vi "Rect Edit.vi"() -> ()   [LabVIEW 2019]
uses:
  Classes/Settings/Rectangle Settings/Rectangle Settings.lvclass/Rectangle Settings.ctl
  typedefs/Schedule Types/Schedule--Constant.ctl
  Classes/Settings/ObjectSettings/ObjectSettings.lvclass/ObjectSettings.ctl
  Classes/Settings/Setting Database/Setting Database.lvclass
  Classes/Settings/Rectangle Settings/Rectangle Settings.lvclass
  C:/Users/Albro/Documents/GitHub/AFM-Lithography/lvsrc/Classes/Settings/ObjectSettings/ObjectSettings.lvclass
  Classes/Settings/Setting Database/Typedefs/PrivateEvents--Setting Database.SetDefaultRectangle.ctl
  Classes/Settings/Setting Database/Typedefs/PrivateEvents--Setting Database.CopyActiveRectangleToAll.ctl
  <vilib>/JKI/JKI SMO/SMO/SMO.lvclass
  Classes/Settings/Rectangle Settings/Accessors/Write Fill Spacing.vi
  Classes/Settings/ObjectSettings/Accessors/Read Voltage Settings.vi
  Classes/Settings/ObjectSettings/Accessors/Read Speed Settings.vi
  Classes/Settings/ObjectSettings/Accessors/Write Resistance.vi
  Classes/Settings/ObjectSettings/Accessors/Write Speed Schedule.vi
  Classes/Settings/ObjectSettings/Accessors/Write Voltage Schedule.vi
  Classes/Settings/ObjectSettings/Accessors/Write Direction.vi
  Classes/Settings/ObjectSettings/Accessors/Write Enabled.vi
  Classes/Settings/Rectangle Settings/Accessors/Write Fill Orientation.vi
  Classes/Settings/ObjectSettings/Accessors/Read Enabled.vi
  Classes/Settings/ObjectSettings/Accessors/Read Direction.vi
  Classes/Settings/Rectangle Settings/Accessors/Read Fill Orientation.vi
  Classes/Settings/Rectangle Settings/Accessors/Read Fill Spacing.vi
  Classes/Settings/ObjectSettings/Accessors/Read Speed Schedule.vi
  Classes/Settings/ObjectSettings/Accessors/Read Voltage Schedule.vi
  Classes/Settings/ObjectSettings/Accessors/Read Resistance.vi
  Classes/Settings/ObjectSettings/ObjectSettings.lvclass
panel:
  in  "Save Default":bool
  in  "Set Resistance":T1(ring) caption="Enum"
  in  "Copy to All":bool
  in  "Speed Settings":bool
  in  "Speed (um/s)":dbl caption="Numeric 2"
  in  "Voltage Settings":bool
  in  "Voltage (V)":dbl caption="Numeric 2"
  in  "Fill Spacing":dbl caption="Numeric 2"
  in  "Voltage Schedule":u16(ring) caption="Ring" items=["Constant", "Ramp", "Fn. Generator", "Formula"]
  in  "Fill Orientation":u16(ring) caption="Ring" items=["Horizontal", "Vertical"]
  in  "Speed Schedule":u16(ring) caption="Ring" items=["Constant", "Ramp", "Fn. Generator", "Formula"]
  in  "Direction":u16(ring) caption="Ring" items=["Forward", "Backward"]
  in  "Index":i32=8
  in  "Enabled?":bool=TRUE
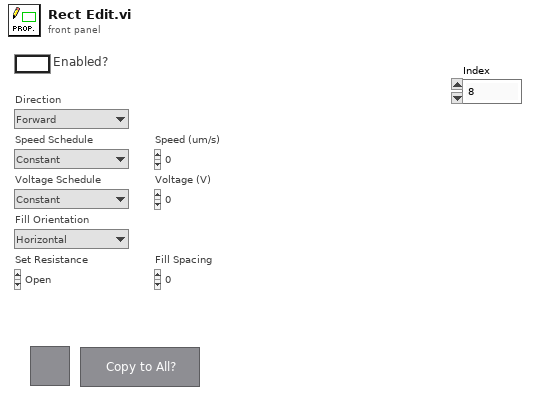
[diagram p1: front panel]
types:
  T1 = enum16{"Open", "Discharge Tip", "0 ohm", "100 kohm", "10 Mohm", "1 Gohm"}
  T2 = typedef "Schedule--Constant.ctl" = cluster{"Value":dbl}
  T3 = enum32{"invalid app kind", "Development System", "Run Time System", "Student Edition", "Embedded LabVIEW", "Evaluation", "Custom"}
  T4 = enum8{"Enabled", "Disabled", "Disabled and Grayed Out"}
  T5 = enum32{"Invalid", "Standard", "Closed", "Hidden", "Minimized", "Maximized"}
  T6 = typedef "Setting Database.lvclass/PrivateEvents--Setting Database.SetDefaultRectangle.ctl" = bool
  T7 = typedef "Setting Database.lvclass/PrivateEvents--Setting Database.CopyActiveRectangleToAll.ctl" = bool
  T8 = typedef "Setting Database.lvclass/PublicEvents--Setting Database.NewActiveRectangle.ctl" = refnum<class "Rectangle Settings.lvclass">
  T9 = cluster{"Core":cluster{"Current VI Reference":refnum<vi>, "Close Panel on Exit?":bool}, "SettingDB":refnum<class "Setting Database.lvclass">, "Rectangle Settings":refnum<class "Rectangle Settings.lvclass">}
  T10 = cluster{"Current VI Reference":refnum<vi>, "Close Panel on Exit?":bool}
  T11 = typedef "Setting Database.lvclass/PublicEvents--Cluster.ctl" = cluster{"NewActivePath":refnum<user-event>, "PathsUpdated":refnum<user-event>, "RectanglesUpdated":refnum<user-event>, "NewActiveRectangle":refnum<user-event>, "NewActiveFunnel":refnum<user-event>, "FunnelsUpdated":refnum<user-event>, "NewActiveDot":refnum<user-event>, "DotsUpdated":refnum<user-event>}
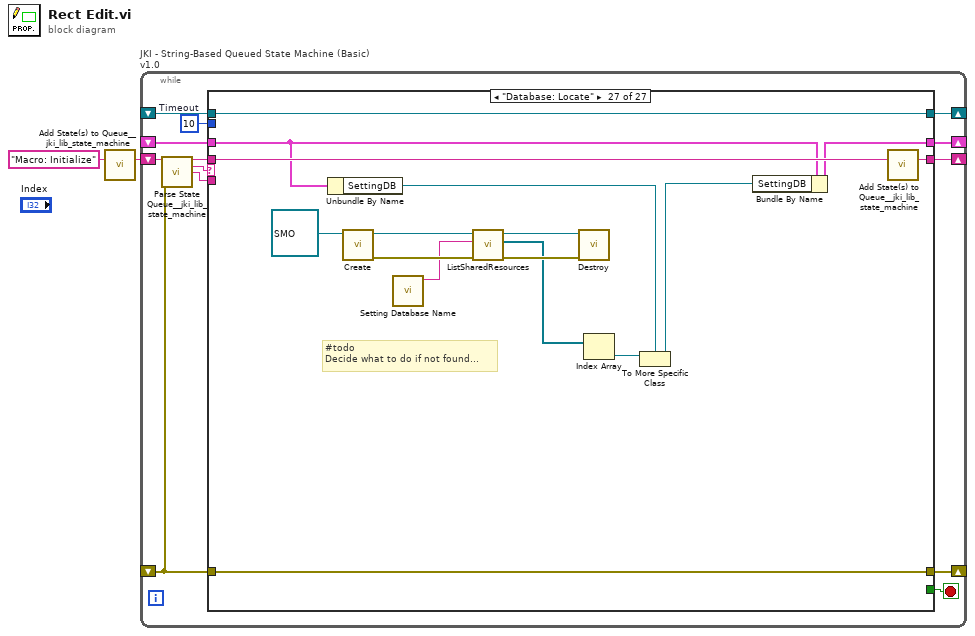
[diagram p0: block diagram]
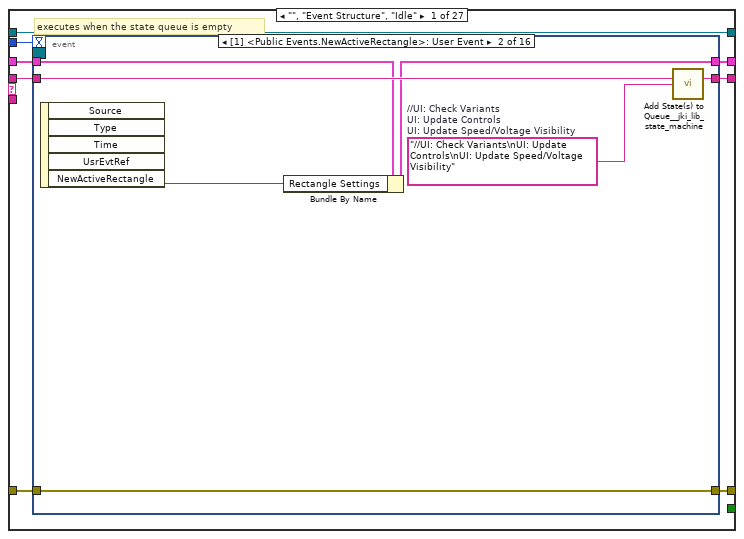
[diagram p2: hidden frame]
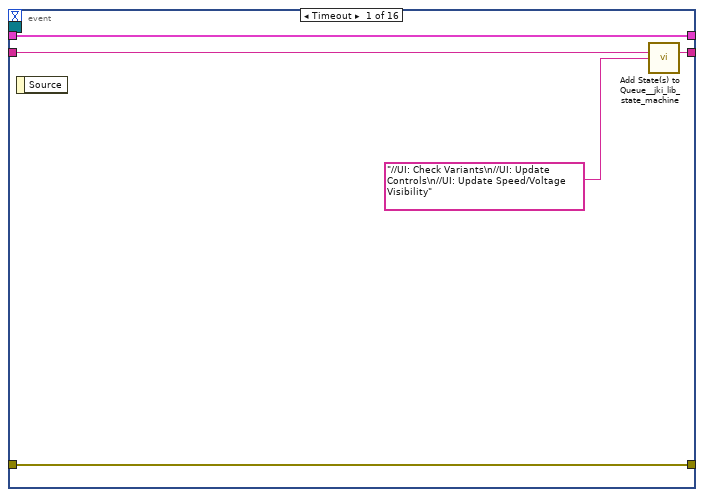
[diagram p3: hidden frame]
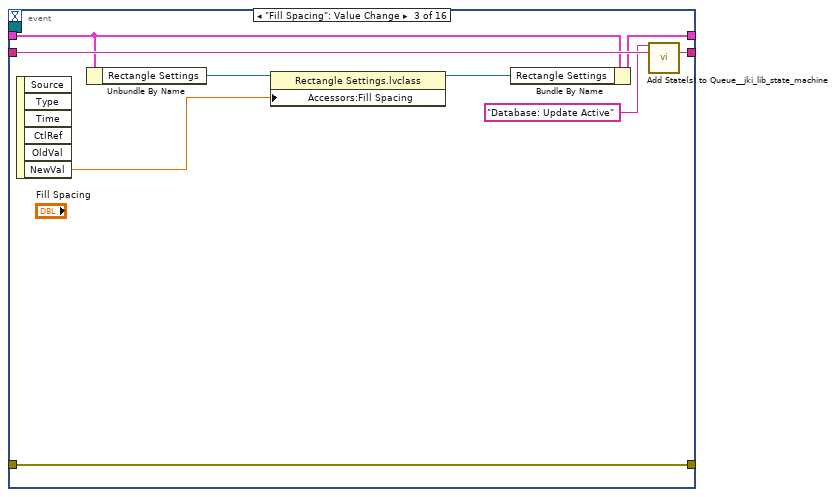
[diagram p4: hidden frame]
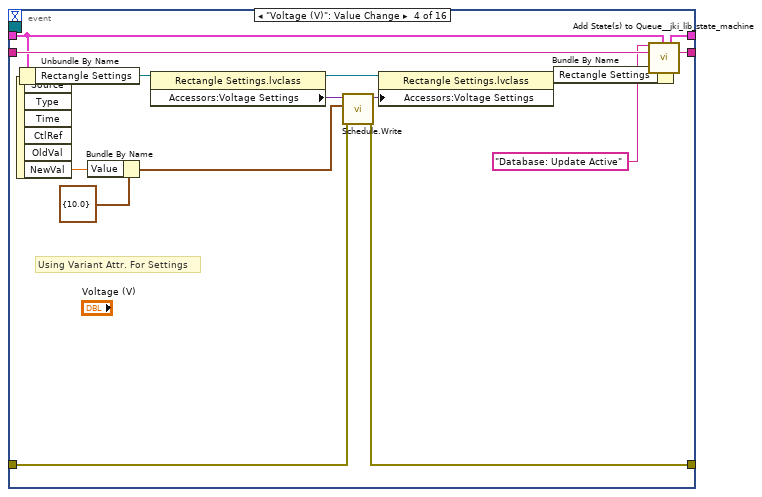
[diagram p5: hidden frame]
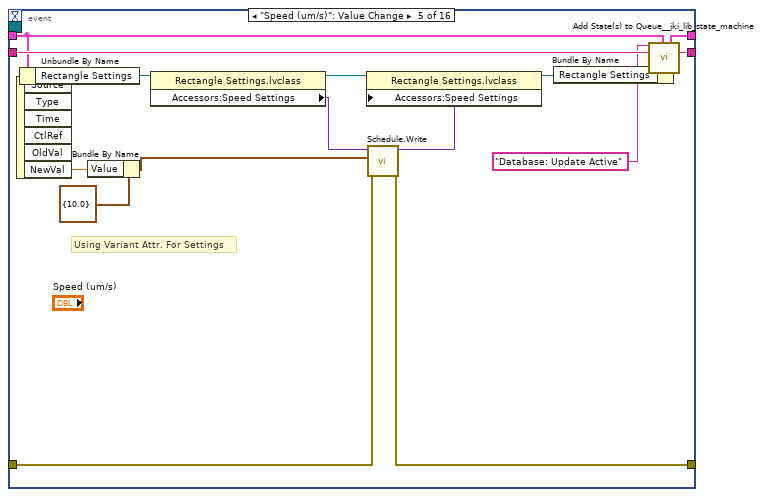
[diagram p6: hidden frame]
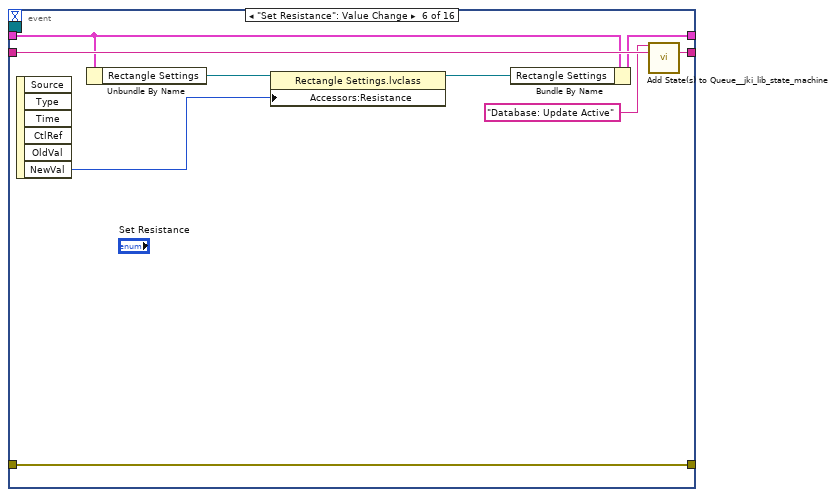
[diagram p7: hidden frame]
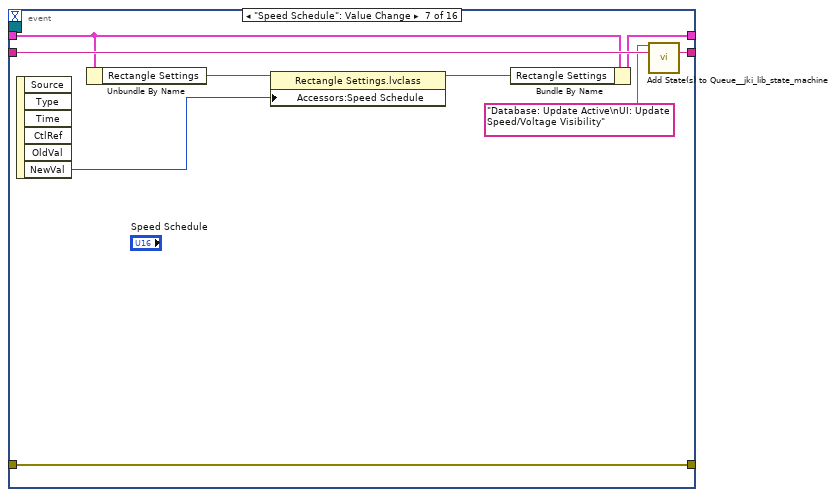
[diagram p8: hidden frame]
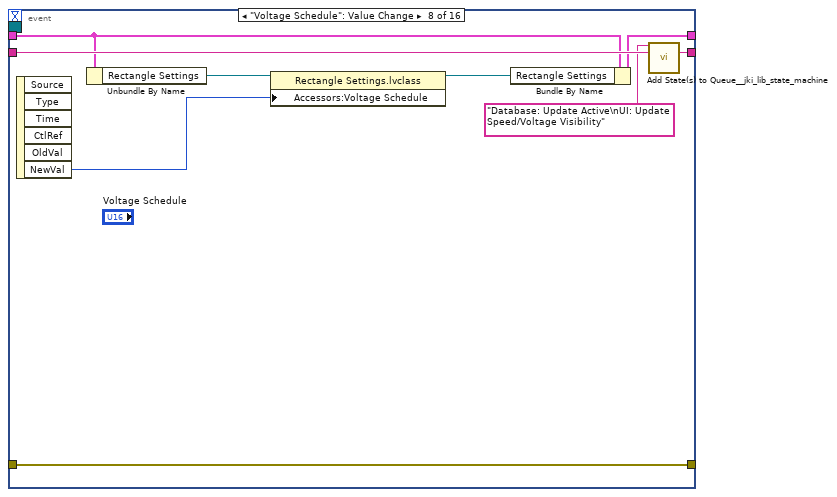
[diagram p9: hidden frame]
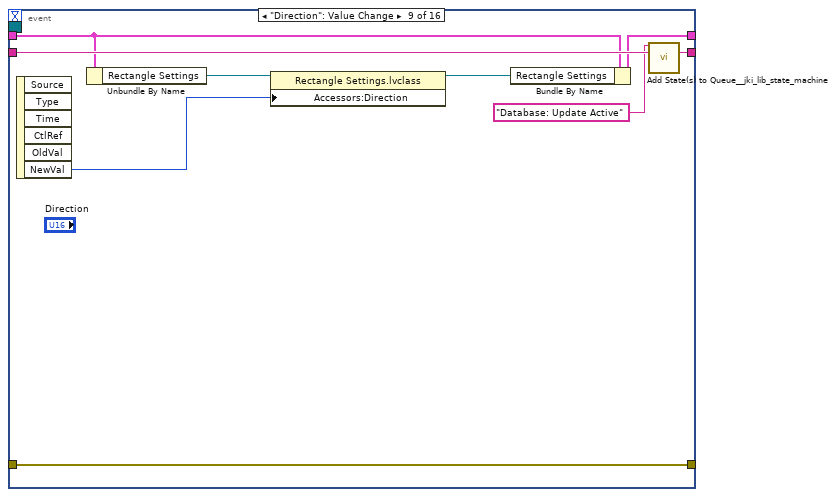
[diagram p10: hidden frame]
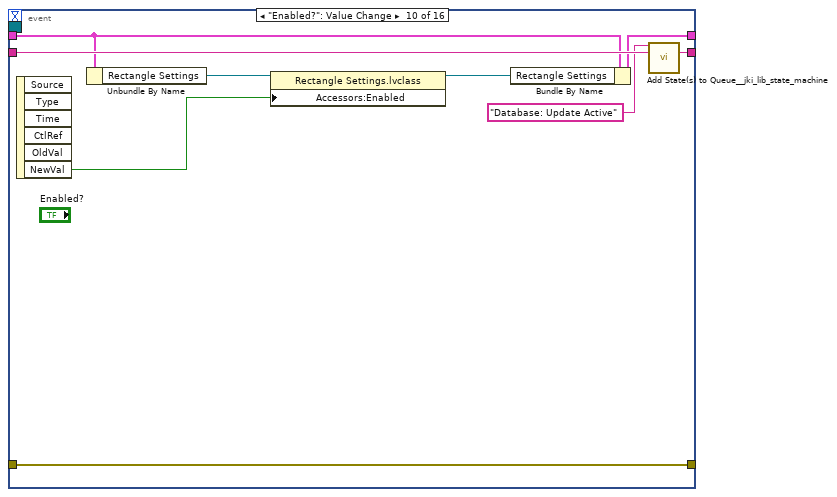
[diagram p11: hidden frame]
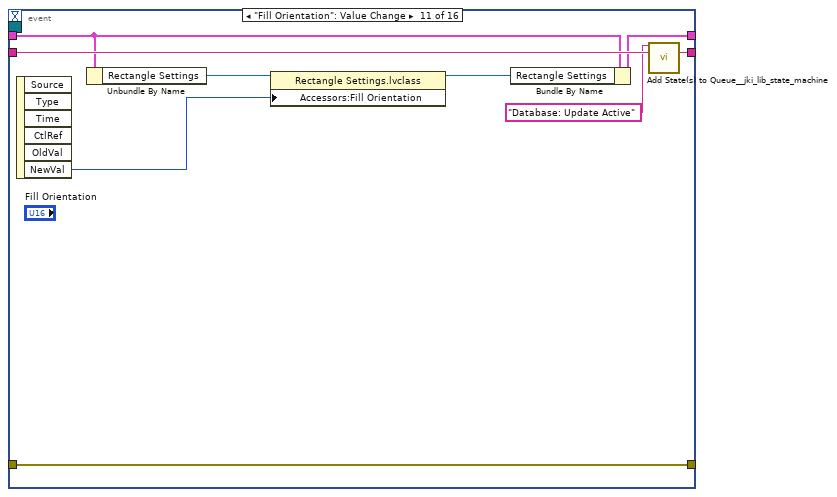
[diagram p12: hidden frame]
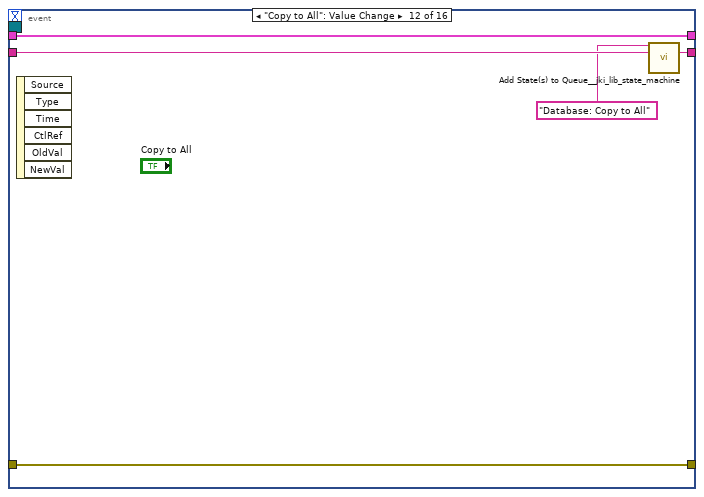
[diagram p13: hidden frame]
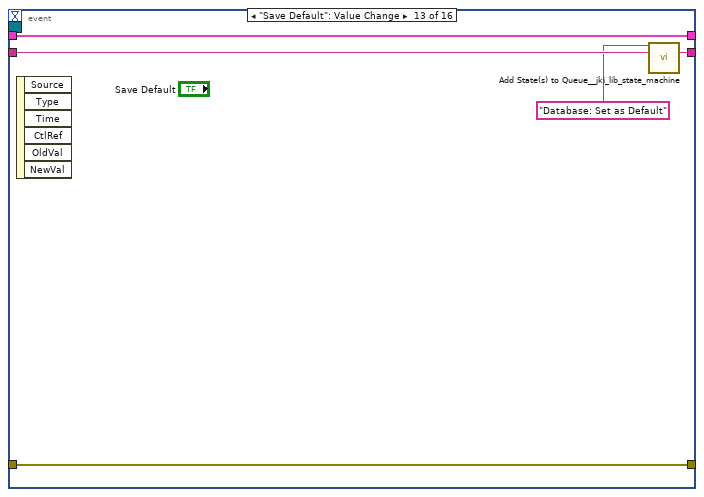
[diagram p14: hidden frame]
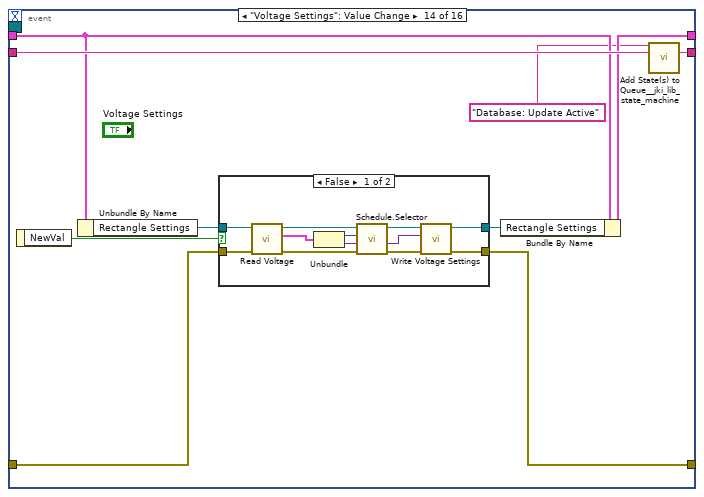
[diagram p15: hidden frame]
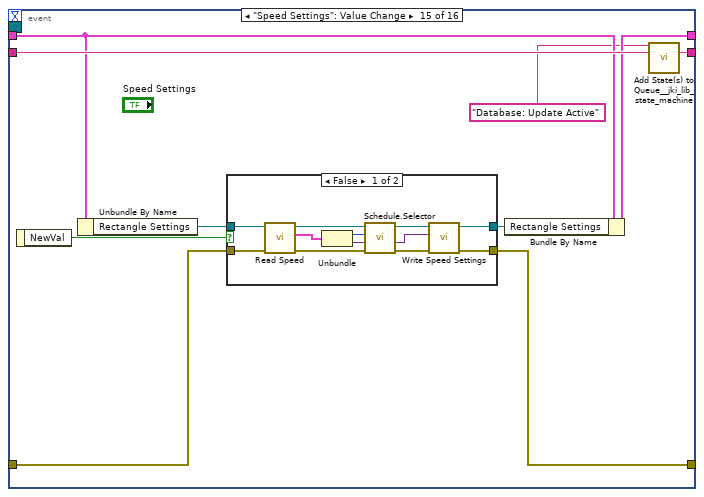
[diagram p17: hidden frame]
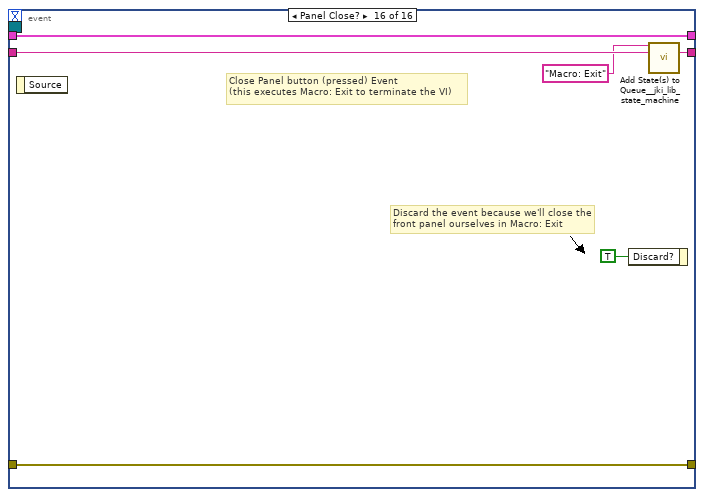
[diagram p19: hidden frame]
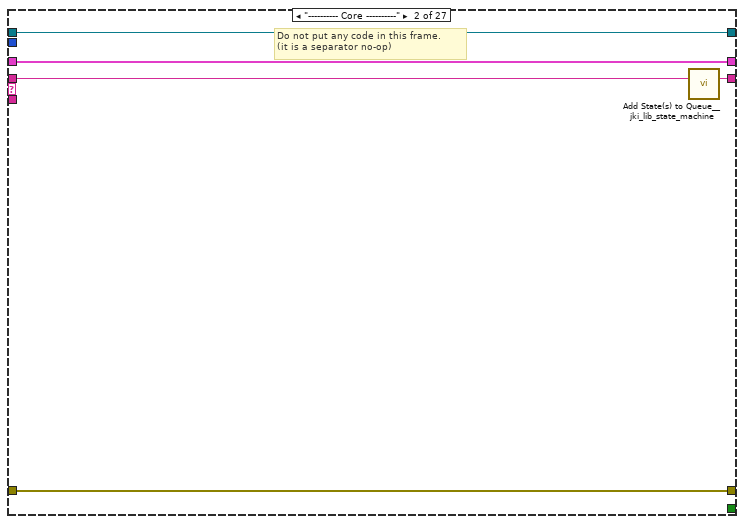
[diagram p20: hidden frame]
diagram:
  n1 = call <vilib>:"Add State(s) to Queue__jki_lib_state_machine.vi"("State(s) in (\"\")"="Macro: Initialize") -> ("States Out"=w2:string)  [unwired: 14 in]
  n2 = while "JKI - String-Based Queued State Machine (Basic) v1.0" {
    shift-right: [w8] -> _
    shift-left: _ -> [w7]
    shift-right: [w11] -> _
    shift-left: _ -> [w5]
    shift-right: [w10] -> _
    shift-left: w2 -> [w12]
    shift-right: [w4] -> _
    shift-left: _ -> [w3]
    stop <- w9 stop-if-true
    w6 = 10  # Timeout
    n3 = call <vilib>:"Parse State Queue__jki_lib_state_machine.vi"("State Queue"=w12, "Error In (no error)"=w5) -> ("Remaining States"=w14:string, "Current State"=w15:string, "Arguments"=w13:string)  [unwired: 11 in]
    n4 = case shown="\"Database: Locate\"" w15 {
      selector: w15 -> [_ _ w203 _ _ _ _ _ _ _ _ _ _ _ _ _ _ _ _ _ _ _ _ _ _ _ _]
      tunnel: w14 -> [w23 w197 w201 w222 w229 w235 w240 w248 w255 w260 w270 w276 w281 w296 w304 w328 w335 w354 w366 w393 w399 w410 w415 w425 w435 w445 w461]
      tunnel: w13 -> [_ _ _ _ _ _ _ _ _ _ _ _ _ _ _ _ w331 _ w360 _ _ _ _ _ _ _ _]
      tunnel: w7 -> [w21 w194 w202 w215 w224 w231 w237 _ w252 w257 w266 w274 w278 w289 w302 w322 w330 w352 w361 w390 w395 w401 w411 w421 w431 w441 w448]
      tunnel: [w20 w195 w206 w220 errorcluster {"status"=FALSE, "code"=0, "source"=""} ("error out") w233 w238 w244 w250 w258 w265 w271 w279 w293 w298 w326 w332 w345 w363 w391 w397 w408 w413 w418 w427 w438 w459] -> w11
      tunnel: w5 -> [w19 w195 w205 w220 w226 w233 w238 w244 w251 w258 w264 w272 w279 w292 w297 w326 w333 w348 w364 w391 w397 w408 w413 w417 w426 w437 w459]
      tunnel: [w22 w196 w204 w221 w228 w234 w239 w247 w254 w259 w269 w275 w280 w295 w303 w327 w334 w353 w365 w392 w398 w409 w414 w424 w434 w444 w460] -> w10
      tunnel: [_ _ _ _ _ TRUE _ _ _ _ _ _ _ _ _ _ _ _ _ _ _ _ _ _ _ _ _] -> w9
      tunnel: [w18 w194 w202 w214 w224 w231 w237 w246 w252 w257 w266 w274 w278 w290 w302 w322 w330 w352 w361 w390 w395 w401 w411 w422 w432 w442 w449] -> w8
      tunnel: w6 -> [w17 _ _ _ _ _ _ _ _ _ _ _ _ _ _ _ _ _ _ _ _ _ _ _ _ _ _]
      tunnel: [w16 w193 w198 w210 w223 w230 w236 w243 w249 w256 w268 w273 w277 w291 w301 w323 w329 w340 w359 w389 w394 w400 w412 w423 w433 w443 w458] -> w4
      tunnel: w3 -> [w16 w193 w198 w210 w223 w230 w236 w243 w249 w256 _ w273 w277 w291 w301 w323 w329 w340 w359 w389 w394 w400 w412 w423 w433 w443 w458]
      frame "", "Event Structure", "Idle" {
        # "executes when the state queue is empty"
        n5 = event shown="[1] <Public Events.NewActiveRectangle>: User Event" {
          selector: w16 -> [_ _ _ _ _ _ _ _ _ _ _ _ _ _ _ _]
          dyn-events: _ -> [_ _ _ _ _ _ _ _ _ _ _ _ _ _ _ _]
          timeout: w17 -> [_ _ _ _ _ _ _ _ _ _ _ _ _ _ _ _]
          tunnel: w23 -> [w28 w35 w44 w59 w74 w83 w92 w101 w110 w119 w128 w133 w138 w148 w172 w192]
          tunnel: [w27 w34 w43 w58 w73 w82 w91 w100 w109 w118 w127 w132 w137 w147 w171 w191] -> w22
          tunnel: w21 -> [w25 w31 w39 w55 w70 w78 w87 w96 w105 w114 w123 w131 w136 w145 w169 w189]
          tunnel: [w26 w33 w42 w46 w62 w81 w90 w99 w108 w117 w126 w130 w135 w142 w165 w190] -> w20
          tunnel: w19 -> [w26 w33 w42 w47 w60 w81 w90 w99 w108 w117 w126 w130 w135 w141 w163 w190]
          tunnel: [w25 w32 w41 w57 w72 w80 w89 w98 w107 w116 w125 w131 w136 w146 w170 w189] -> w18
          event Timeout {
            n6 = event-data() -> ()  [unwired: 1 in, 1 out]
            n7 = call <vilib>:"Add State(s) to Queue__jki_lib_state_machine.vi"("State(s) in (\"\")"=w28, "State(s) at Back (\"\")"="//UI: Check Variants\n//UI: Update Controls\n//UI: Update Speed/Voltage Visibility") -> ("States Out"=w27:string)  [unwired: 13 in]
          }
          event User Event {
            w29 = "//UI: Check Variants\nUI: Update Controls\nUI: Update Speed/Voltage Visibility"  # //UI: Check Variants UI: Update Controls UI: Update Speed/Voltage Visibility
            n8 = event-data() -> ("NewActiveRectangle"=w30:T8)  [unwired: 1 in, 4 out]
            n9 = Bundle By Name(cluster=w31, "Rectangle Settings"=w30) -> (w32:T9)
            n10 = call <vilib>:"Add State(s) to Queue__jki_lib_state_machine.vi"("State(s) in (\"\")"=w35, "State(s) at Back (\"\")"=w29) -> ("States Out"=w34:string)  [unwired: 13 in]
          }
          event "Fill Spacing": Value Change {
            n11 = event-data() -> ("NewVal"=w37:dbl)  [unwired: 1 in, 5 out]
            n12 = Unbundle By Name(w39) -> ("Rectangle Settings"=w40:refnum<class "Rectangle Settings.lvclass">)
            n13 = property class="Rectangle Settings.lvclass"(reference=w40, "Accessors:Fill Spacing"=w37) -> (reference out=w38:refnum<class "Rectangle Settings.lvclass">)  [unwired: 1 in, 1 out]
            n14 = Bundle By Name(cluster=w39, "Rectangle Settings"=w38) -> (w41:T9)
            n15 = call <vilib>:"Add State(s) to Queue__jki_lib_state_machine.vi"("State(s) in Front (\"\")"="Database: Update Active", "State(s) in (\"\")"=w44) -> ("States Out"=w43:string)  [unwired: 13 in]
          }
          event "Voltage (V)": Value Change {
            # "Using Variant Attr. For Settings"
            n16 = event-data() -> ("NewVal"=w50:dbl)  [unwired: 1 in, 5 out]
            n17 = Unbundle By Name(w55) -> ("Rectangle Settings"=w56:refnum<class "Rectangle Settings.lvclass">)
            n18 = Bundle By Name(cluster=T2 {"Value"=10.0} ("Constant"), "Value"=w50) -> (w45:T2)
            n19 = property class="Rectangle Settings.lvclass"(reference=w56) -> (reference out=w54:refnum<class "Rectangle Settings.lvclass">, "Accessors:Voltage Settings"=w49:variant)  [unwired: 1 in, 1 out]
            n20 = call "Schedule.Write.vi"("error in (no error)"=w47, "Data to Write"=w45, "LUT In"=w49) -> ("error out"=w46:errorcluster, "LUT Out"=w48:variant)  [unwired: 7 in]
            n21 = property class="Rectangle Settings.lvclass"(reference=w54, "Accessors:Voltage Settings"=w48) -> (reference out=w52:refnum<class "Rectangle Settings.lvclass">)  [unwired: 1 in, 1 out]
            n22 = Bundle By Name(cluster=w55, "Rectangle Settings"=w52) -> (w57:T9)
            n23 = call <vilib>:"Add State(s) to Queue__jki_lib_state_machine.vi"("State(s) in Front (\"\")"="Database: Update Active", "State(s) in (\"\")"=w59) -> ("States Out"=w58:string)  [unwired: 13 in]
          }
          event "Speed (um/s)": Value Change {
            # "Using Variant Attr. For Settings"
            n24 = event-data() -> ("NewVal"=w65:dbl)  [unwired: 1 in, 5 out]
            n25 = Unbundle By Name(w70) -> ("Rectangle Settings"=w71:refnum<class "Rectangle Settings.lvclass">)
            n26 = Bundle By Name(cluster=T2 {"Value"=10.0} ("Constant"), "Value"=w65) -> (w61:T2)
            n27 = property class="Rectangle Settings.lvclass"(reference=w71) -> (reference out=w69:refnum<class "Rectangle Settings.lvclass">, "Accessors:Speed Settings"=w64:variant)  [unwired: 1 in, 1 out]
            n28 = call "Schedule.Write.vi"("error in (no error)"=w60, "Data to Write"=w61, "LUT In"=w64) -> ("error out"=w62:errorcluster, "LUT Out"=w63:variant)  [unwired: 7 in]
            n29 = property class="Rectangle Settings.lvclass"(reference=w69, "Accessors:Speed Settings"=w63) -> (reference out=w67:refnum<class "Rectangle Settings.lvclass">)  [unwired: 1 in, 1 out]
            n30 = Bundle By Name(cluster=w70, "Rectangle Settings"=w67) -> (w72:T9)
            n31 = call <vilib>:"Add State(s) to Queue__jki_lib_state_machine.vi"("State(s) in Front (\"\")"="Database: Update Active", "State(s) in (\"\")"=w74) -> ("States Out"=w73:string)  [unwired: 13 in]
          }
          event "Set Resistance": Value Change {
            n32 = event-data() -> ("NewVal"=w76:T1)  [unwired: 1 in, 5 out]
            n33 = Unbundle By Name(w78) -> ("Rectangle Settings"=w79:refnum<class "Rectangle Settings.lvclass">)
            n34 = property class="Rectangle Settings.lvclass"(reference=w79, "Accessors:Resistance"=w76) -> (reference out=w77:refnum<class "Rectangle Settings.lvclass">)  [unwired: 1 in, 1 out]
            n35 = Bundle By Name(cluster=w78, "Rectangle Settings"=w77) -> (w80:T9)
            n36 = call <vilib>:"Add State(s) to Queue__jki_lib_state_machine.vi"("State(s) in Front (\"\")"="Database: Update Active", "State(s) in (\"\")"=w83) -> ("States Out"=w82:string)  [unwired: 13 in]
          }
          event "Speed Schedule": Value Change {
            n37 = event-data() -> ("NewVal"=w85:u16)  [unwired: 1 in, 5 out]
            n38 = Unbundle By Name(w87) -> ("Rectangle Settings"=w88:refnum<class "Rectangle Settings.lvclass">)
            n39 = property class="Rectangle Settings.lvclass"(reference=w88, "Accessors:Speed Schedule"=w85) -> (reference out=w86:refnum<class "Rectangle Settings.lvclass">)  [unwired: 1 in, 1 out]
            n40 = Bundle By Name(cluster=w87, "Rectangle Settings"=w86) -> (w89:T9)
            n41 = call <vilib>:"Add State(s) to Queue__jki_lib_state_machine.vi"("State(s) in Front (\"\")"="Database: Update Active\nUI: Update Speed/Voltage Visibility", "State(s) in (\"\")"=w92) -> ("States Out"=w91:string)  [unwired: 13 in]
          }
          event "Voltage Schedule": Value Change {
            n42 = event-data() -> ("NewVal"=w94:u16)  [unwired: 1 in, 5 out]
            n43 = Unbundle By Name(w96) -> ("Rectangle Settings"=w97:refnum<class "Rectangle Settings.lvclass">)
            n44 = property class="Rectangle Settings.lvclass"(reference=w97, "Accessors:Voltage Schedule"=w94) -> (reference out=w95:refnum<class "Rectangle Settings.lvclass">)  [unwired: 1 in, 1 out]
            n45 = Bundle By Name(cluster=w96, "Rectangle Settings"=w95) -> (w98:T9)
            n46 = call <vilib>:"Add State(s) to Queue__jki_lib_state_machine.vi"("State(s) in Front (\"\")"="Database: Update Active\nUI: Update Speed/Voltage Visibility", "State(s) in (\"\")"=w101) -> ("States Out"=w100:string)  [unwired: 13 in]
          }
          event "Direction": Value Change {
            n47 = event-data() -> ("NewVal"=w103:u16)  [unwired: 1 in, 5 out]
            n48 = Unbundle By Name(w105) -> ("Rectangle Settings"=w106:refnum<class "Rectangle Settings.lvclass">)
            n49 = property class="Rectangle Settings.lvclass"(reference=w106, "Accessors:Direction"=w103) -> (reference out=w104:refnum<class "Rectangle Settings.lvclass">)  [unwired: 1 in, 1 out]
            n50 = Bundle By Name(cluster=w105, "Rectangle Settings"=w104) -> (w107:T9)
            n51 = call <vilib>:"Add State(s) to Queue__jki_lib_state_machine.vi"("State(s) in Front (\"\")"="Database: Update Active", "State(s) in (\"\")"=w110) -> ("States Out"=w109:string)  [unwired: 13 in]
          }
          event "Enabled?": Value Change {
            n52 = event-data() -> ("NewVal"=w112:bool)  [unwired: 1 in, 5 out]
            n53 = Unbundle By Name(w114) -> ("Rectangle Settings"=w115:refnum<class "Rectangle Settings.lvclass">)
            n54 = property class="Rectangle Settings.lvclass"(reference=w115, "Accessors:Enabled"=w112) -> (reference out=w113:refnum<class "Rectangle Settings.lvclass">)  [unwired: 1 in, 1 out]
            n55 = Bundle By Name(cluster=w114, "Rectangle Settings"=w113) -> (w116:T9)
            n56 = call <vilib>:"Add State(s) to Queue__jki_lib_state_machine.vi"("State(s) in Front (\"\")"="Database: Update Active", "State(s) in (\"\")"=w119) -> ("States Out"=w118:string)  [unwired: 13 in]
          }
          event "Fill Orientation": Value Change {
            n57 = event-data() -> ("NewVal"=w121:u16)  [unwired: 1 in, 5 out]
            n58 = Unbundle By Name(w123) -> ("Rectangle Settings"=w124:refnum<class "Rectangle Settings.lvclass">)
            n59 = property class="Rectangle Settings.lvclass"(reference=w124, "Accessors:Fill Orientation"=w121) -> (reference out=w122:refnum<class "Rectangle Settings.lvclass">)  [unwired: 1 in, 1 out]
            n60 = Bundle By Name(cluster=w123, "Rectangle Settings"=w122) -> (w125:T9)
            n61 = call <vilib>:"Add State(s) to Queue__jki_lib_state_machine.vi"("State(s) in Front (\"\")"="Database: Update Active", "State(s) in (\"\")"=w128) -> ("States Out"=w127:string)  [unwired: 13 in]
          }
          event "Copy to All": Value Change {
            n62 = event-data() -> ()  [unwired: 1 in, 6 out]
            n63 = call <vilib>:"Add State(s) to Queue__jki_lib_state_machine.vi"("State(s) in Front (\"\")"="Database: Copy to All", "State(s) in (\"\")"=w133) -> ("States Out"=w132:string)  [unwired: 13 in]
          }
          event "Save Default": Value Change {
            n64 = event-data() -> ()  [unwired: 1 in, 6 out]
            n65 = call <vilib>:"Add State(s) to Queue__jki_lib_state_machine.vi"("State(s) in Front (\"\")"="Database: Set as Default", "State(s) in (\"\")"=w138) -> ("States Out"=w137:string)  [unwired: 13 in]
          }
          event "Voltage Settings": Value Change {
            n66 = event-data() -> ("NewVal"=w140:bool)  [unwired: 1 in]
            n67 = Unbundle By Name(w145) -> ("Rectangle Settings"=w143:refnum<class "Rectangle Settings.lvclass">)
            n68 = case shown="False" w140 {
              tunnel: w143 -> [w160 w162]
              tunnel: [w152 w162] -> w144
              tunnel: w141 -> [w159 w161]
              tunnel: [w149 w161] -> w142
              frame False {
                n69 = call "Read Voltage.vi"("error in (no error)"=w159, "ObjectSettings in"=w160) -> ("error out"=w157:errorcluster, "Voltage"=w156:cluster{"Schedule":u16, "Settings":variant}, "ObjectSettings out"=w158:refnum<class "Rectangle Settings.lvclass">)  [unwired: 7 in]
                n70 = Unbundle(w156) -> ("Schedule"=w155:u16, "Settings"=w154:variant)
                n71 = call-dynamic "Schedule.Selector.vi"("error in (no error)"=w157, "Settings In"=w154, "Schedule"=w155, "ObjectSettings in"=w158) -> ("error out"=w151:errorcluster, "Settings Out"=w150:variant, "ObjectSettings out"=w153:refnum<class "Rectangle Settings.lvclass">)  [unwired: 5 in]
                n72 = call "Write Voltage Settings.vi"("error in (no error)"=w151, "Settings"=w150, "ObjectSettings in"=w153) -> ("error out"=w149:errorcluster, "ObjectSettings out"=w152:refnum<class "Rectangle Settings.lvclass">)  [unwired: 7 in]
              }
              frame True {
              }
            }
            n73 = Bundle By Name(cluster=w145, "Rectangle Settings"=w144) -> (w146:T9)
            n74 = call <vilib>:"Add State(s) to Queue__jki_lib_state_machine.vi"("State(s) in Front (\"\")"="Database: Update Active", "State(s) in (\"\")"=w148) -> ("States Out"=w147:string)  [unwired: 13 in]
          }
          event "Speed Settings": Value Change {
            n75 = event-data() -> ("NewVal"=w164:bool)  [unwired: 1 in]
            n76 = Unbundle By Name(w169) -> ("Rectangle Settings"=w167:refnum<class "Rectangle Settings.lvclass">)
            n77 = case shown="False" w164 {
              tunnel: w167 -> [w182 w186]
              tunnel: [w176 w186] -> w166
              tunnel: w163 -> [w180 w185]
              tunnel: [w175 w185] -> w165
              frame False {
                n78 = call "Read Speed.vi"("error in (no error)"=w180, "ObjectSettings in"=w182) -> ("error out"=w179:errorcluster, "Speed"=w178:cluster{"Schedule":u16, "Settings":variant}, "ObjectSettings out"=w181:refnum<class "Rectangle Settings.lvclass">)  [unwired: 7 in]
                n79 = Unbundle(w178) -> ("Schedule"=w184:u16, "Settings"=w183:variant)
                n80 = call-dynamic "Schedule.Selector.vi"("error in (no error)"=w179, "Settings In"=w183, "Schedule"=w184, "ObjectSettings in"=w181) -> ("error out"=w174:errorcluster, "Settings Out"=w173:variant, "ObjectSettings out"=w177:refnum<class "Rectangle Settings.lvclass">)  [unwired: 5 in]
                n81 = call "Write Speed Settings.vi"("error in (no error)"=w174, "Settings"=w173, "ObjectSettings in"=w177) -> ("error out"=w175:errorcluster, "ObjectSettings out"=w176:refnum<class "Rectangle Settings.lvclass">)  [unwired: 7 in]
              }
              frame True {
              }
            }
            n82 = Bundle By Name(cluster=w169, "Rectangle Settings"=w166) -> (w170:T9)
            n83 = call <vilib>:"Add State(s) to Queue__jki_lib_state_machine.vi"("State(s) in Front (\"\")"="Database: Update Active", "State(s) in (\"\")"=w172) -> ("States Out"=w171:string)  [unwired: 13 in]
          }
          event Panel Close? {
            # "Discard the event because we'll close the front panel ourselves in Macro: Exit"
            # "Close Panel button (pressed) Event\n(this executes Macro: Exit to terminate the VI)"
            n84 = event-data() -> ()  [unwired: 1 in, 1 out]
            n85 = event-data("Discard?"=TRUE) -> ()  [unwired: 1 in, 1 out]
            n86 = call <vilib>:"Add State(s) to Queue__jki_lib_state_machine.vi"("State(s) in Front (\"\")"="Macro: Exit", "State(s) in (\"\")"=w192) -> ("States Out"=w191:string)  [unwired: 13 in]
          }
        }
      }
      frame "---------- Core ----------" {
        # "Do not put any code in this frame.\n(it is a separator no-op)"
        n87 = call <vilib>:"Add State(s) to Queue__jki_lib_state_machine.vi"("State(s) in (\"\")"=w197) -> ("States Out"=w196:string)  [unwired: 14 in]
      }
      frame Default {
        w209 = 42 items=["No error", "Argument error", "Memory is full", "Out of zone", "End of file", "File already open", "Generic file I/O error", "File not found", "File permission error", "Disk is full", "Duplicate path", "Too many files open", "System feature not enabled", "Resource file not found", "Cannot add resource", "Resource not found", "Image not found", "Image memory error", "Pen does not exist", "Config type invalid", "Config token not found", "Config parse error", "Config memory error", "Bad external code format", "Bad external code offset", "External code not present", "Null window", "Destroy window error", "Null menu", "Print aborted", "Bad print record", "Print driver error", "Windows error during printing", "Memory error during printing", "Print dialog error", "Generic print error", "Invalid device refnum", "Device not found", "Device parameter error", "Device unit error", "Cannot open device", "Device call aborted", "Generic error", "Cancelled by user", "Object ID too low", "Object ID too high", "Object not in heap", "Unknown heap", "Unknown object (invalid DefProc)", "Unknown object (DefProc not in table)", "Message out of range", "Invalid (null) method", "Unknown message", "Manager call not supported", "Bad address", "Network operation in progress", "Network operation timed out", "Connection is busy", "Network attribute not supported", "Network error", "Address in use", "System out of memory", "Connection aborted", "Connection refused", "Not connected", "Already connected", "Connection closed", "Initialization error (interapplication manager)", "Bad occurrence", "Wait on unbound occurrence handler", "Occurrence queue overflow", "Datalog type conflict", "Unused", "Unrecognized type (interapplication manager)", "Memory corrupt", "Failed to make temporary DLL", "Old CIN version", "Drag socket not found", "Failed to load drop-object", "Failed to register OLE object", "Failed to release OLE object", "Format specifier type mismatch", "Unknown format specifier", "Too few format specifiers", "Too many format specifiers", "Scan failed", "Newer CIN version", "Error converting to variant", "Runtime menu error", "Password tampered", "Variant attribute not found", "Incompatible variant data type", "Event data is not available", "Event Store is not present", "Occurrence is not found", "Event Queue is not created", "Event info is not available", "Refnum passed is NULL", "Error retrieving Class GUID", "Error retrieving CoClass GUID", "Error retrieving TypeLib GUID.", "Bad built application magic bytes.", "Specific driver is different from the specific driver associated with the Logical Name.", "There is no session opened to the class driver.", "Max Error", "MAX - Error with config objects", "MAX - Error loading configuration", "MAX - Group not supported"]
        # "Current State"
        # "Do not delete, rename, or modify this frame.\n(this is used to capture unhandled states and typos)"
        # "Handle mistyped state name (developer tool)"
        n88 = Format Into String(format string="Software Exception: Unhandled State \"%s\"." ("message"), error in=w205, w203) -> (resulting string=w208:string, error out=w207:errorcluster)  [unwired: 1 in]
        n89 = call <vilib>:"Error Cluster From Error Code.vi"("show call chain? (False)"=TRUE, "error in (no error)"=w207, "error message (\"\")"=w208, "error code (0)"=w209) -> ("error out"=w206:errorcluster)  [unwired: 5 in]
        n90 = call <vilib>:"Add State(s) to Queue__jki_lib_state_machine.vi"("State(s) in (\"\")"=w201) -> ("States Out"=w204:string)  [unwired: 14 in]
      }
      frame "Initialize Core Data" {
        # "exe?"
        # "If panel starts closed or is an EXE, then close it when we exit"
        # "Do not delete, rename, or modify this frame.\n(this is used to determine panel behavior on exit)"
        n91 = property class="VI"() -> ("Front Panel.Open"=w218:bool)  [unwired: 2 in, 2 out]
        n92 = property class="App"() -> ("App.Kind"=w217:T3)  [unwired: 2 in, 2 out]
        n93 = control-ref of="Current VI Reference"() -> (w219:refnum<vi>)
        n94 = Not(x=w218) -> (.not. x?=w213:bool)
        n95 = Equal?(x=w217, y=T3."Run Time System" ("Application:Kind")) -> (x = y?=w212:bool)
        n96 = Or(x=w213, y=w212) -> (x .or. y?=w216:bool)
        n97 = Bundle By Name(cluster=w215, "Core.Current VI Reference"=w219, "Core.Close Panel on Exit?"=w216) -> (w214:T9)
        n98 = call <vilib>:"Add State(s) to Queue__jki_lib_state_machine.vi"("State(s) in (\"\")"=w222) -> ("States Out"=w221:string)  [unwired: 14 in]
      }
      frame "Error Handler" {
        # "Unhandled Error -- Display it"
        # "Handle any errors here.\nYou can also output any states to clean-up after errors occur"
        # "Clear error"
        n99 = call <vilib>:"General Error Handler.vi"("error in (no error)"=w226) -> ()  [unwired: 10 in, 5 out]
        n100 = call <vilib>:"Add State(s) to Queue__jki_lib_state_machine.vi"("State(s) in Front (\"\")"="/* Post Error States", "State(s) in (\"\")"=w229) -> ("States Out"=w228:string)  [unwired: 13 in]
      }
      frame "Exit" {
        # "Do not put any code in this frame.\n(No errors that occur here will be handled.)"
        n101 = call <vilib>:"Add State(s) to Queue__jki_lib_state_machine.vi"("State(s) in (\"\")"=w235) -> ("States Out"=w234:string)  [unwired: 14 in]
      }
      frame "---------- Data ----------" {
        # "Do not put any code in this frame.\n(It is a separator no-op. You can make a copy of this frame to create a new Data frame)"
        n102 = call <vilib>:"Add State(s) to Queue__jki_lib_state_machine.vi"("State(s) in (\"\")"=w240) -> ("States Out"=w239:string)  [unwired: 14 in]
      }
      frame "Data: Initialize" {
        w241 = refnum<class "Rectangle Settings.lvclass"> refnum  # Rectangle Settings
        w242 = refnum<class "Setting Database.lvclass"> refnum  # SettingDB
        w245 = T10 {"Current VI Reference"=refnum, "Close Panel on Exit?"=FALSE}  # Core
        # "Initialize the shift-register data, here.\n(data names are defined by what you wire into the bundle function)"
        n103 = Bundle("Core"=w245, "SettingDB"=w242, "Rectangle Settings"=w241) -> (w246:T9)  [unwired: 1 in]
        n104 = call <vilib>:"Add State(s) to Queue__jki_lib_state_machine.vi"("State(s) in (\"\")"=w248) -> ("States Out"=w247:string)  [unwired: 14 in]
      }
      frame "Data: Cleanup" {
        # "Cleanup any data and references, here.\n(this is called automatically, by the Macro: Exit)"
        n105 = Unbundle By Name(w252) -> ("Core.Current VI Reference"=w253:refnum<vi>)
        n106 = Close Reference(reference=w253, error in (no error)=w251) -> (error out=w250:errorcluster)
        n107 = call <vilib>:"Add State(s) to Queue__jki_lib_state_machine.vi"("State(s) in (\"\")"=w255) -> ("States Out"=w254:string)  [unwired: 14 in]
      }
      frame "---------- Events ----------" {
        # "Do not put any code in this frame.\n(It is a separator no-op. You can make a copy of this frame to create a new UI frame)"
        n108 = call <vilib>:"Add State(s) to Queue__jki_lib_state_machine.vi"("State(s) in (\"\")"=w260) -> ("States Out"=w259:string)  [unwired: 14 in]
      }
      frame "Events: Register" {
        # "Do not put any code in this frame.\n(It is a separator no-op. You can make a copy of this frame to create a new UI frame)"
        n109 = Unbundle By Name(w266) -> ("SettingDB"=w263:refnum<class "Setting Database.lvclass">)
        n110 = call "Setting Database.GetPublicEvents.vi"("Setting Database"=w263) -> ("error out"=w261:errorcluster, "Public Events"=w262:T11)  [unwired: 8 in, 1 out]
        n111 = register-events(w262) -> (reference out=w268:refnum<event-registration>, error out=w267:errorcluster)  [unwired: 2 in]
        n112 = Merge Errors(w264, w267, w261) -> (w265:errorcluster)
        n113 = call <vilib>:"Add State(s) to Queue__jki_lib_state_machine.vi"("State(s) in (\"\")"=w270) -> ("States Out"=w269:string)  [unwired: 14 in]
      }
      frame "Events: Unregister" {
        # "Do not put any code in this frame.\n(It is a separator no-op. You can make a copy of this frame to create a new UI frame)"
        n114 = Unregister For Events(event registration refnum=w273, error in=w272) -> (error out=w271:errorcluster)
        n115 = call <vilib>:"Add State(s) to Queue__jki_lib_state_machine.vi"("State(s) in (\"\")"=w276) -> ("States Out"=w275:string)  [unwired: 14 in]
      }
      frame "---------- UI ----------" {
        # "Do not put any code in this frame.\n(It is a separator no-op. You can make a copy of this frame to create a new UI frame)"
        n116 = call <vilib>:"Add State(s) to Queue__jki_lib_state_machine.vi"("State(s) in (\"\")"=w281) -> ("States Out"=w280:string)  [unwired: 14 in]
      }
      frame "UI: Check Variants" {
        # "Do not put any code in this frame.\n(It is a separator no-op. You can make a copy of this frame to create a new UI frame)"
        n117 = Unbundle By Name(w289) -> ("Rectangle Settings"=w288:refnum<class "Rectangle Settings.lvclass">)
        n118 = property class="Rectangle Settings.lvclass"(reference=w288) -> (reference out=w287:refnum<class "Rectangle Settings.lvclass">, "Accessors:Voltage Settings"=w285:variant, "Accessors:Speed Settings"=w283:variant)  [unwired: 1 in, 1 out]
        n119 = call "Schedule.CheckVariantAttributes.vi"("error in (no error)"=w292, "Variant In"=w283) -> ("error out"=w294:errorcluster, "Variant Out"=w282:variant)  [unwired: 8 in]
        n120 = call "Schedule.CheckVariantAttributes.vi"("error in (no error)"=w294, "Variant In"=w285) -> ("error out"=w293:errorcluster, "Variant Out"=w284:variant)  [unwired: 8 in]
        n121 = property class="Rectangle Settings.lvclass"(reference=w287, "Accessors:Voltage Settings"=w284, "Accessors:Speed Settings"=w282) -> (reference out=w286:refnum<class "Rectangle Settings.lvclass">)  [unwired: 1 in, 1 out]
        n122 = Bundle By Name(cluster=w289, "Rectangle Settings"=w286) -> (w290:T9)
        n123 = call <vilib>:"Add State(s) to Queue__jki_lib_state_machine.vi"("State(s) in (\"\")"=w296) -> ("States Out"=w295:string)  [unwired: 14 in]
      }
      frame "UI: Initialize" {
        # "Initialize the User Interface, here.\n(this is called automatically, by the Macro: Init)"
        n124 = control-ref of="Speed Schedule"() -> (w300:refnum<vi>)
        n125 = property class="Ring (strict)"(reference=w300, error in=w297, "DisabledEnum"=T4."Disabled and Grayed Out" ("Disabled")) -> (error out=w298:errorcluster)  [unwired: 1 out]
        n126 = call <vilib>:"Add State(s) to Queue__jki_lib_state_machine.vi"("State(s) in (\"\")"=w304) -> ("States Out"=w303:string)  [unwired: 14 in]
      }
      frame "UI: Update Controls" {
        w311 = T2 {"Value"=10.0} ("Constant")
        # "Using Variant Attr. For Settings"
        n127 = Unbundle By Name(w322) -> ("Rectangle Settings"=w321:refnum<class "Rectangle Settings.lvclass">)
        n128 = property class="Rectangle Settings.lvclass"(reference=w321) -> ("Accessors:Enabled"=w320:bool, "Accessors:Direction"=w319:u16, "Accessors:Fill Orientation"=w318:u16, "Accessors:Fill Spacing"=w317:dbl, "Accessors:Speed Schedule"=w316:u16, "Accessors:Voltage Schedule"=w315:u16, "Accessors:Resistance"=w314:T1, "Accessors:Speed Settings"=w308:variant, "Accessors:Voltage Settings"=w306:variant)  [unwired: 1 in, 2 out]
        n129 = local write "Enabled?"(w320) -> ()
        n130 = local write "Fill Orientation"(w318) -> ()
        n131 = local write "Speed Schedule"(w316) -> ()
        n132 = local write "Set Resistance"(w314) -> ()
        n133 = call "Schedule.CheckVariantAttributes.vi"("Variant In"=w308) -> ("Variant Out"=w307:variant)  [unwired: 9 in, 1 out]
        n134 = call "Schedule.CheckVariantAttributes.vi"("Variant In"=w306) -> ("Variant Out"=w305:variant)  [unwired: 9 in, 1 out]
        n135 = call "Schedule.Read.vi"("Data to Read"=w311, "LUT In"=w307) -> ("Data Out"=w313:variant)  [unwired: 7 in, 2 out]
        n136 = call "Schedule.Read.vi"("Data to Read"=w311, "LUT In"=w305) -> ("Data Out"=w310:variant)  [unwired: 7 in, 2 out]
        n137 = local write "Direction"(w319) -> ()
        n138 = local write "Voltage Schedule"(w315) -> ()
        n139 = local write "Fill Spacing"(w317) -> ()
        n140 = Variant To Data(type=w311, Variant=w313) -> (data=w312:T2)  [unwired: 1 in, 1 out]
        n141 = Variant To Data(type=w311, Variant=w310) -> (data=w309:T2)  [unwired: 1 in, 1 out]
        n142 = Unbundle(w312) -> ("Value"=w325:dbl)
        n143 = Unbundle(w309) -> ("Value"=w324:dbl)
        n144 = local write "Speed (um/s)"(w325) -> ()
        n145 = local write "Voltage (V)"(w324) -> ()
        n146 = call <vilib>:"Add State(s) to Queue__jki_lib_state_machine.vi"("State(s) in (\"\")"=w328) -> ("States Out"=w327:string)  [unwired: 14 in]
      }
      frame "UI: Cursor Set" {
        # "Argument"
        # "Set and Unset Cursor Busy.\n(Usage: \"UI: Cursor Set >> Busy|Idle\")"
        n147 = case shown="\"Idle\", Default" w331 {
          tunnel: w333 -> [w337 w339]
          tunnel: [w336 w338] -> w332
          frame "Idle", Default {
            n148 = call <vilib>:"Unset Busy.vi"("error in (no error)"=w337) -> ("error out"=w336:errorcluster)  [unwired: 10 in]
          }
          frame "Busy" {
            n149 = call <vilib>:"Set Busy.vi"("error in (no error)"=w339) -> ("error out"=w338:errorcluster)  [unwired: 9 in, 1 out]
          }
        }
        n150 = call <vilib>:"Add State(s) to Queue__jki_lib_state_machine.vi"("State(s) in (\"\")"=w335) -> ("States Out"=w334:string)  [unwired: 14 in]
      }
      frame "UI: Update Speed/Voltage Visibility" {
        n151 = local read "Voltage Schedule"() -> (w350:u16)
        n152 = local read "Speed Schedule"() -> (w351:u16)
        n153 = case shown="0" w350 {
          tunnel: [TRUE FALSE] -> w347
          frame 0 {
          }
          frame 1, Default {
          }
        }
        n154 = case shown="0" w351 {
          tunnel: [TRUE FALSE] -> w349
          frame 0 {
          }
          frame 1, Default {
          }
        }
        n155 = property on="Voltage (V)" class="DigNum (strict)"(error in=w348, "Visible"=w347) -> (error out=w342:errorcluster)  [unwired: 1 in, 1 out]
        n156 = Not(x=w347) -> (.not. x?=w343:bool)
        n157 = property on="Voltage Settings" class="Bool (strict)"(error in=w342, "Visible"=w343) -> (error out=w341:errorcluster)  [unwired: 1 in, 1 out]
        n158 = property on="Speed (um/s)" class="DigNum (strict)"(error in=w341, "Visible"=w349) -> (error out=w344:errorcluster)  [unwired: 1 in, 1 out]
        n159 = Not(x=w349) -> (.not. x?=w346:bool)
        n160 = property on="Speed Settings" class="Bool (strict)"(error in=w344, "Visible"=w346) -> (error out=w345:errorcluster)  [unwired: 1 in, 1 out]
        n161 = call <vilib>:"Add State(s) to Queue__jki_lib_state_machine.vi"("State(s) in (\"\")"=w354) -> ("States Out"=w353:string)  [unwired: 14 in]
      }
      frame "UI: Front Panel State" {
        # "Argument"
        # "Set Front Panel Open or Closed\n(Usage: \"UI: Front Panel State >> Open|Close\")"
        n162 = Unbundle By Name(w361) -> ("Core.Current VI Reference"=w362:refnum<vi>)
        n163 = case shown="\"Open\", Default" w360 {
          tunnel: w364 -> [w370 w383]
          tunnel: [w372 w384] -> w363
          tunnel: w362 -> [w371 w381]
          frame "Open", Default {
            n164 = property class="VI"(reference=w371, error in=w370) -> (reference out=w368:refnum<vi>, error out=w369:errorcluster, "Front Panel.Open"=w367:bool)
            n165 = case shown="False" w367 {
              tunnel: [w375 w378] -> w372
              tunnel: w369 -> [w374 w378]
              tunnel: w368 -> [w373 _]
              frame False {
                n166 = invoke class="VI" method="FP.Open"(reference=w373, error in=w374, "Activate"=TRUE, "State"=T5."Standard") -> (error out=w375:errorcluster)  [unwired: 1 in, 4 out]
              }
              frame True {
              }
            }
          }
          frame "Close" {
            n167 = property class="VI"(reference=w381, error in=w383) -> (reference out=w380:refnum<vi>, error out=w382:errorcluster, "Front Panel.Open"=w379:bool)
            n168 = case shown="True" w379 {
              tunnel: [w385 w388] -> w384
              tunnel: w382 -> [w385 w387]
              tunnel: w380 -> [_ w386]
              frame False {
              }
              frame True {
                n169 = invoke class="VI" method="FP.Close"(reference=w386, error in=w387) -> (error out=w388:errorcluster)  [unwired: 1 in, 2 out]
              }
            }
          }
        }
        n170 = call <vilib>:"Add State(s) to Queue__jki_lib_state_machine.vi"("State(s) in (\"\")"=w366) -> ("States Out"=w365:string)  [unwired: 14 in]
      }
      frame "---------- Macro ----------" {
        # "Do not put any code in this frame.\n(It is a separator no-op. You can make a copy of this frame to create a new Macro frame)"
        n171 = call <vilib>:"Add State(s) to Queue__jki_lib_state_machine.vi"("State(s) in (\"\")"=w393) -> ("States Out"=w392:string)  [unwired: 14 in]
      }
      frame "Macro: Initialize" {
        # "Initialization Macro\n(This is called once, when the VI starts)"
        n172 = call <vilib>:"Add State(s) to Queue__jki_lib_state_machine.vi"("State(s) in Front (\"\")"="Data: Initialize\nInitialize Core Data\nDatabase: Locate\nEvents: Register\nUI: Initialize\n//UI: Check Variants\n//UI: Update Controls\nUI: Update Speed/Voltage Visibility\nUI: Front Panel State >> Close", "State(s) in (\"\")"=w399) -> ("States Out"=w398:string)  [unwired: 13 in]
      }
      frame "Macro: Exit" {
        # "Exit Macro\n(This is called once, when the VI exits)"
        n173 = Unbundle By Name(w401) -> ("Core.Close Panel on Exit?"=w407:bool)
        n174 = Select(t="UI: Front Panel State >> Close", s=w407, f="") -> (s? t:f=w404:string)
        n175 = call <vilib>:"Add State(s) to Queue__jki_lib_state_machine.vi"("State(s) in (\"\")"=w404, "State(s) at Back (\"\")"="Data: Cleanup\nEvents: Unregister\nExit") -> ("States Out"=w402:string)  [unwired: 13 in]
        n176 = call <vilib>:"Add State(s) to Queue__jki_lib_state_machine.vi"("State(s) in Front (\"\")"=w402, "State(s) in (\"\")"=w410) -> ("States Out"=w409:string)  [unwired: 13 in]
      }
      frame "---------- Database ----------" {
        n177 = call <vilib>:"Add State(s) to Queue__jki_lib_state_machine.vi"("State(s) in (\"\")"=w415) -> ("States Out"=w414:string)  [unwired: 14 in]
      }
      frame "Database: Set as Default" {
        n178 = Unbundle By Name(w421) -> ("SettingDB"=w420:refnum<class "Setting Database.lvclass">)
        n179 = call "Setting Database.SetDefaultRectangle.vi"("error in (no error)"=w417, "SetDefaultRectangle"=T6 TRUE, "Setting Database"=w420) -> ("error out"=w418:errorcluster, "Setting Database out"=w419:refnum<class "Setting Database.lvclass">)  [unwired: 7 in]
        n180 = Bundle By Name(cluster=w421, "SettingDB"=w419) -> (w422:T9)
        n181 = call <vilib>:"Add State(s) to Queue__jki_lib_state_machine.vi"("State(s) in (\"\")"=w425) -> ("States Out"=w424:string)  [unwired: 14 in]
      }
      frame "Database: Update Active" {
        n182 = Unbundle By Name(w431) -> ("SettingDB"=w430:refnum<class "Setting Database.lvclass">, "Rectangle Settings"=w428:refnum<class "Rectangle Settings.lvclass">)
        n183 = call "Setting Database.UpdateActiveRectangle.vi"("error in (no error)"=w426, "UpdateActiveRectangle"=w428, "Setting Database"=w430) -> ("error out"=w427:errorcluster, "Setting Database"=w429:refnum<class "Setting Database.lvclass">)  [unwired: 7 in]
        n184 = Bundle By Name(cluster=w431, "SettingDB"=w429) -> (w432:T9)
        n185 = call <vilib>:"Add State(s) to Queue__jki_lib_state_machine.vi"("State(s) in (\"\")"=w435) -> ("States Out"=w434:string)  [unwired: 14 in]
      }
      frame "Database: Copy to All" {
        n186 = Unbundle By Name(w441) -> ("SettingDB"=w440:refnum<class "Setting Database.lvclass">)
        n187 = call "Setting Database.CopyActiveRectangleToAll.vi"("error in (no error)"=w437, "CopyActiveRectangleToAll"=T7 TRUE, "Setting Database"=w440) -> ("error out"=w438:errorcluster, "Setting Database out"=w439:refnum<class "Setting Database.lvclass">)  [unwired: 7 in]
        n188 = Bundle By Name(cluster=w441, "SettingDB"=w439) -> (w442:T9)
        n189 = call <vilib>:"Add State(s) to Queue__jki_lib_state_machine.vi"("State(s) in (\"\")"=w445) -> ("States Out"=w444:string)  [unwired: 14 in]
      }
      frame "Database: Locate" {
        # "#todo\nDecide what to do if not found..."
        n190 = Unbundle By Name(w448) -> ("SettingDB"=w450:refnum<class "Setting Database.lvclass">)
        n191 = call <vilib>:"Create.vi"("SMO"=refnum<class "SMO.lvclass"> refnum) -> ("error out"=w455:errorcluster, "SMO out"=w457:refnum<class "SMO.lvclass">)  [unwired: 8 in, 1 out]
        n192 = call "Setting Database Name.vi"() -> ("Name"=w453:string)  [unwired: 10 in, 1 out]
        n193 = call <vilib>:"ListSharedResources.vi"("error in (no error)"=w455, "Filter (regex|name)"=w453, "SMO in"=w457) -> ("error out"=w454:errorcluster, "Shared Resources"=w452:refnum<class "SMO.lvclass">[], "SMO out"=w456:refnum<class "SMO.lvclass">)  [unwired: 5 in, 1 out]
        n194 = call <vilib>:"Destroy.vi"("error in (no error)"=w454, "SMO"=w456) -> ()  [unwired: 9 in, 1 out]
        n195 = Index Array(array=w452) -> (element=w451:refnum<class "SMO.lvclass">)  [unwired: 1 in]
        n196 = To More Specific Class(target class=w450, reference=w451) -> (specific class reference=w447:refnum<class "Setting Database.lvclass">)  [unwired: 1 in, 1 out]
        n197 = Bundle By Name(cluster=w448, "SettingDB"=w447) -> (w449:T9)
        n198 = call <vilib>:"Add State(s) to Queue__jki_lib_state_machine.vi"("State(s) in (\"\")"=w461) -> ("States Out"=w460:string)  [unwired: 14 in]
      }
    }
  }
